vi "Excel ActiveX Example.vi"() -> ()   [LabVIEW 2017]
uses:
  <vilib>/regexp/Match Regular Expression.xnode
panel:
  in  "Excel._Worksheet":refnum<k7>
  in  "Excel._Application":refnum<k7>
  # "Overview:This example prompts for a file and for the letter of the column to delete.\nRequirements:\n•\tLabVIEW 2012 (or compatible)\nInstructions:\n•\tRun the program\n•\tSelect the excel file to revise."
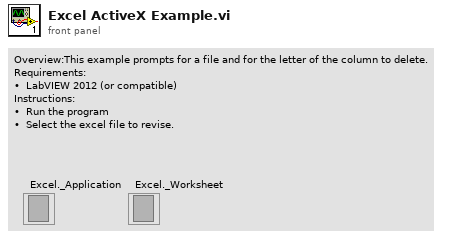
[diagram p1: front panel]
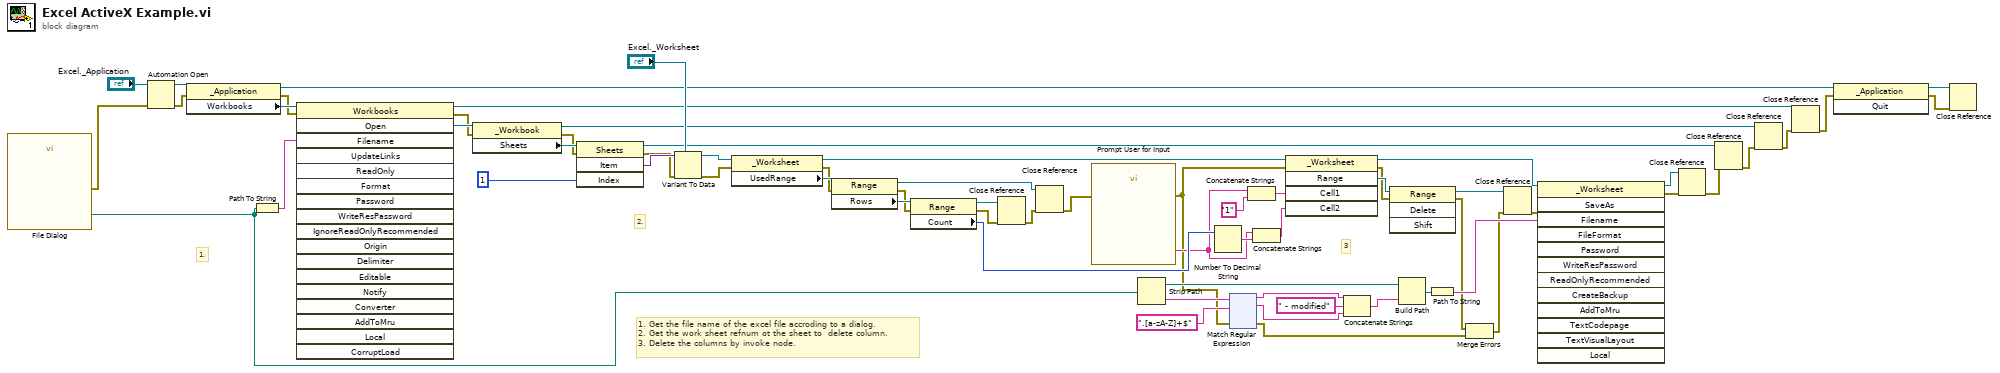
[diagram p0: block diagram]
diagram:
  # "1. Get the file name of the excel file accroding to a dialog.\n2. Get the work sheet refnum ot the sheet to  delete column.\n3. Delete the columns by invoke node."
  # "3"
  # "2."
  # "1."
  n1 = call "File Dialog"() -> ("selected path"=w19:path, "error out"=w5:errorcluster)  [unwired: 12 in, 2 out]
  n2 = Automation Open(error in (no error)=w5, Automation Refnum="Excel._Application") -> (Automation Refnum=w38:refnum<k7>, error out=w37:errorcluster)  [unwired: 2 in]
  n3 = property class="_Application"(reference=w38, error in=w37) -> (reference out=w40:refnum<k7>, error out=w63:errorcluster, "Workbooks"=w64:refnum<k7>)
  n4 = Path To String(path=w19) -> (string=w20:string)
  n5 = invoke class="Workbooks" method="Open"(reference=w64, error in=w63, "Filename"=w20) -> (reference out=w47:refnum<k7>, error out=w50:errorcluster, "Open"=w62:refnum<k7>)  [unwired: 15 in, 15 out]
  n6 = property class="_Workbook"(reference=w62, error in=w50) -> (reference out=w48:refnum<k7>, error out=w51:errorcluster, "Sheets"=w61:refnum<k7>)
  n7 = invoke class="Sheets" method="Item"(reference=w61, error in=w51, "Index"=1) -> (reference out=w49:refnum<k7>, error out=w52:errorcluster, "Item"=w60:variant)  [unwired: 1 in, 1 out]
  n8 = Variant To Data(error in=w52, type="Excel._Worksheet", Variant=w60) -> (data=w33:refnum<k7>, error out=w29:errorcluster)
  n9 = property class="_Worksheet"(reference=w33, error in=w29) -> (reference out=w27:refnum<k7>, error out=w35:errorcluster, "UsedRange"=w36:refnum<k7>)
  n10 = property class="Range"(reference=w36, error in=w35) -> (reference out=w21:refnum<k7>, error out=w28:errorcluster, "Rows"=w34:refnum<k7>)
  n11 = property class="Range"(reference=w34, error in=w28) -> (reference out=w22:refnum<k7>, error out=w24:errorcluster, "Count"=w31:i32)
  n12 = Close Reference(reference=w22, error in (no error)=w24) -> (error out=w23:errorcluster)
  n13 = Close Reference(reference=w21, error in (no error)=w23) -> (error out=w6:errorcluster)
  n14 = call "Prompt User for Input"("error in (no error)"=w6) -> ("Column Letter"=w7:string, "error out"=w4:errorcluster)  [unwired: 16 in, 1 out]
  n15 = Strip Path(path=w19) -> (stripped path=w18:path, name=w15:string)
  n16 = Number To Decimal String(number=w31) -> (decimal integer string=w32:string)  [unwired: 1 in]
  n17 = xnode "Match Regular Expression"("input string"=w15, "regular expression"=".[a-zA-Z]+$", "error in"=w4) -> ("before match"=w13:string, "whole match"=w12:string, "error out"=w3:errorcluster)  [unwired: 3 in, 2 out]
  n18 = Concatenate Strings(w7, "1" ("string")) -> (w8:string)
  n19 = Concatenate Strings(w7, w32) -> (w30:string)
  n20 = invoke class="_Worksheet" method="Range"(reference=w27, error in=w4, "Cell1"=w8, "Cell2"=w30) -> (reference out=w56:refnum<k7>, error out=w53:errorcluster, "Range"=w57:refnum<k7>)  [unwired: 1 in, 2 out]
  n21 = Concatenate Strings(w13, " - modified" ("string"), w12) -> (w11:string)
  n22 = invoke class="Range" method="Delete"(reference=w57, error in=w53) -> (reference out=w55:refnum<k7>, error out=w2:errorcluster)  [unwired: 2 in, 2 out]
  n23 = Build Path(base path=w18, name or relative path=w11) -> (appended path=w17:path)
  n24 = Path To String(path=w17) -> (string=w10:string)
  n25 = Merge Errors(w2, w3) -> (w1:errorcluster)
  n26 = Close Reference(reference=w55, error in (no error)=w1) -> (error out=w54:errorcluster)
  n27 = invoke class="_Worksheet" method="SaveAs"(reference=w56, error in=w54, "Filename"=w10) -> (reference out=w25:refnum<k7>, error out=w26:errorcluster)  [unwired: 10 in, 11 out]
  n28 = Close Reference(reference=w25, error in (no error)=w26) -> (error out=w41:errorcluster)
  n29 = Close Reference(reference=w49, error in (no error)=w41) -> (error out=w42:errorcluster)
  n30 = Close Reference(reference=w48, error in (no error)=w42) -> (error out=w43:errorcluster)
  n31 = Close Reference(reference=w47, error in (no error)=w43) -> (error out=w44:errorcluster)
  n32 = invoke class="_Application" method="Quit"(reference=w40, error in=w44) -> (reference out=w46:refnum<k7>, error out=w45:errorcluster)  [unwired: 1 in, 1 out]
  n33 = Close Reference(reference=w46, error in (no error)=w45) -> ()  [unwired: 1 out]
